vi "AlliGator Run XY Graph Python Function.vi"(6 "AlliGator Ctrl Refnums":T1, 8 "error in (no error)":errorcluster, 9 "Python Function Info":T9={"Script Path"=path "", "Function Name"="", "Function Parent Menu"="", "Function Input Parameters"=[], "Function Outputs"=[], "Function Doc String"="", "Function Display Name"="", "Function Target Type"=enum."Window Menu", "Function Target Window"="", "Parent Menu Location"="", "Item Menu Tag"="", "Is preceded by Separator"=FALSE}, 10 "Mouse Click Event Data":T13, 11 "data value reference in":refnum<data-value>) -> (0 "error out":errorcluster, 1 "Message":string, 3 "Data Value Reference out":refnum<data-value>)   [LabVIEW 2021, in "AlliGator Python Plugins.lvlib"]
doc: "Calls a XY Graph-associated python function."
uses:
  AlliGator Python Plugins.lvlib
  Graphs/XY Graph/XY Graph Mouse Click Event Data.ctl
  Graphs/XY Graph/XY Graph Refnum.ctl
  <vilib>/Utility/miscctls.llb/LVPoint32TypeDef.ctl
  AlliGator Python Function Information.ctl
  AlliGator Python Function Parameter Definition.ctl
  AlliGator Python Function Output Definition.ctl
  AlliGator Python Plugin Target Type.ctl
  AlliGator Internal Variables v2.ctl
  <vilib>/vision/Image Controls.llb/IMAQ Image.ctl
  AlliGator Gate Image Set.ctl
  AlliGator FLI Dataset Type.ctl
  AlliGator Data Series Type.ctl
  AlliGator Dataset Channel.ctl
  AlliGator Gate Arithmetic.ctl
  AlliGator Displayed Image.ctl
  Image/Named ROI Description.ctl
  AlliGator Decay Metadata v3.ctl
  AlliGator Decay Background Subtraction Info.ctl
  AlliGator Baseline Subtraction Method.ctl
  Graphs/XY Graph/XY Graph Plot Shift Parameters.ctl
  Graphs/XY Graph/XY Graph Plot Shift Method.ctl
  AlliGator Decay Extrapolation Parameters.ctl
  Phasor/Calibration Phasor (m, phi).ctl
  Phasor/Phasor Reference Series.ctl
  Phasor/Phasor Calibration Map v2.ctl
  Phasor/Phasor (g, s).ctl
  AlliGator Raw Phasor Plot Data v4.ctl
  Phasor/Phasor Standard Deviation Options.ctl
  AlliGator Phasor Multi-Harmonic Data.ctl
  Phasor/Phasor Harmonic Data.ctl
  AlliGator Decay Fit Options & Parameters v2.ctl
  Fits/IRF(X)PSED/Decay Fit Options v2.ctl
  Fits/Decay Convolution/Decay Model.ctl
  Fits/Residual Type.ctl
  Fits/IRF(X)PSED/Fit Weights Type.ctl
  Fits/Non-linear Fitting Method v2.ctl
  Fits/Fit Calculation Method.ctl
  Fits/Non-linear Fitting Algorithm.ctl
  AlliGator Decay Fit Parameter Constraints 2.ctl
  Fits/IRF(X)PSED/Decay Fit Parameters In List.ctl
  Fits/IRF(X)PSED/MLE Baseline Offset Type.ctl
  AlliGator Decay Preprocessing Parameters.ctl
  Fits/IRF(X)PSED/Decay Fit Parameters & Derived Quantities List.ctl
  AlliGator Ctrl Refnums.ctl
  AlliGator Other Ctrl Refnums.ctl
  AlliGator State Indicator.ctl
  AlliGator Phasor Plot Ctrl Refnums.ctl
  AlliGator Phasor Graph Ctrl Refnums.ctl
  Phasor/Phasor Calibration Type.ctl
  AlliGator Dataset Ctrl Refnums.ctl
  AlliGator Registered Events Ctrl Refnums.ctl
  AlliGator Image Histogram Control Refnums.ctl
  Histograms/Linear Histogram Options.ctl
  Histograms/Histogram Bin Option.ctl
  Histograms/Histogram Bin Position.ctl
  AlliGator Decay Fit Map Control Refnums.ctl
  AlliGator Variables List.ctl
  AlliGator Python Plugin Plot Data.ctl
  AlliGator Python Plugin Graph Data Input.ctl
  Graphs/Get Plot at Mouse Click (XY Graph)/Get Plot at Mouse Click [AAC].vi
  Graphs/XY Graph/XY Graph Add Multiplots with Names.vi
  Graphs/Graphs.lvlib
  Graphs/XY Graph/XY Graph Add-Ons.lvlib
  AlliGator Globals, Variables & Constants.lvlib
  Strings/Strings.lvlib
  Error/Error.lvlib
  AlliGator GUI.lvlib
  Phasor/Phasor.lvlib
  Image/Image.lvlib
  AlliGator Decay Preprocessing.lvlib
  AlliGator Phasor Graph.lvlib
  AlliGator Files.lvlib
  AlliGator Phasor Plot.lvlib
  AlliGator Source Image.lvlib
  Fits/Fits.lvlib
  AlliGator Decay Fit.lvlib
  AlliGator Decay Fit Parameter Map.lvlib
  AlliGator Settings.lvlib
  AlliGator Internal Variables.lvlib
  AlliGator Dual-Channel Datasets.lvlib
  Histograms/Histogram Window.lvlib
panel:
  out "Function Parameters String":string
  # "see the AlliGator License on the block diagram (Ctrl+E or Window:Show Block Diagram)"
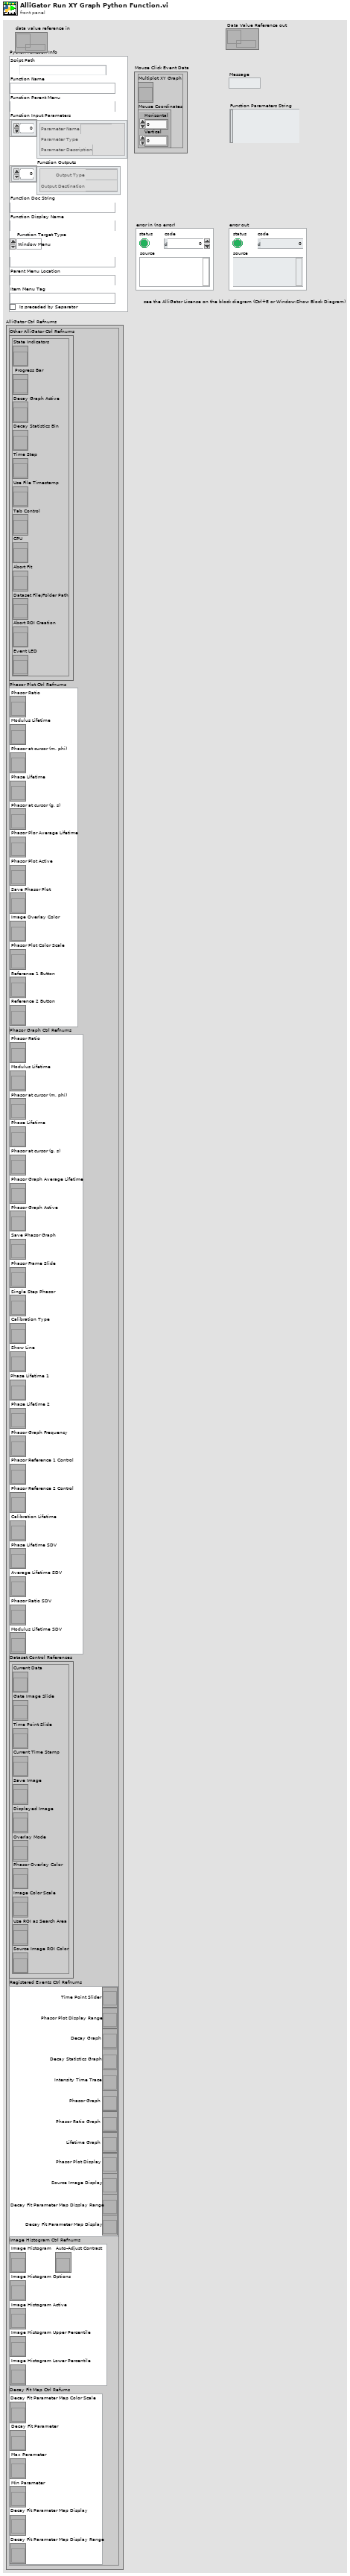
[diagram p1: front panel]
types:
  T1 = typedef "AlliGator GUI.lvlib/AlliGator Ctrl Refnums.ctl" = cluster{"Other AlliGator Ctrl Refnums":T2, "Phasor Plot Ctrl Refnums":T3, "Phasor Graph Ctrl Refnums":T4, "Dataset Control References":T5, "Registered Events Ctrl Refnums":T6, "Image Histogram Ctrl Refnums":T7, "Decay Fit Map Ctrl Refums":T8}
  T2 = typedef "AlliGator GUI.lvlib/AlliGator Other Ctrl Refnums.ctl" = cluster{"State Indicators":refnum<vi>, " Progress Bar":refnum<vi>, "Decay Graph Active":refnum<vi>, "Decay Statistics Bin":refnum<vi>, "Time Step":refnum<vi>, "Use File Timestamp":refnum<vi>, "Tab Control":refnum<vi>, "CPU":refnum<vi>, "Abort Fit":refnum<vi>, "Dataset File/Folder Path":refnum<vi>, "Abort ROI Creation":refnum<vi>, "Event LED":refnum<vi>}
  T3 = typedef "AlliGator GUI.lvlib/AlliGator Phasor Plot Ctrl Refnums.ctl" = cluster{"Phasor Ratio":refnum<vi>, "Modulus Lifetime":refnum<vi>, "Phasor at cursor (m, phi)":refnum<vi>, "Phase Lifetime":refnum<vi>, "Phasor at cursor (g, s)":refnum<vi>, "Phasor Plor Average Lifetime":refnum<vi>, "Phasor Plot Active":refnum<vi>, "Save Phasor Plot":refnum<vi>, "Image Overlay Color":refnum<vi>, "Phasor Plot Color Scale":refnum<vi>, "Reference 1 Button":refnum<vi>, "Reference 2 Button":refnum<vi>}
  T4 = typedef "AlliGator GUI.lvlib/AlliGator Phasor Graph Ctrl Refnums.ctl" = cluster{"Phasor Ratio":refnum<vi>, "Modulus Lifetime":refnum<vi>, "Phasor at cursor (m, phi)":refnum<vi>, "Phase Lifetime":refnum<vi>, "Phasor at cursor (g, s)":refnum<vi>, "Phasor Graph Average Lifetime":refnum<vi>, "Phasor Graph Active":refnum<vi>, "Save Phasor Graph":refnum<vi>, "Phasor Frame Slide":refnum<vi>, "Single Step Phasor":refnum<vi>, "Calibration Type":refnum<vi>, "Show Line":refnum<vi>, "Phase Lifetime 1":refnum<vi>, "Phase Lifetime 2":refnum<vi>, "Phasor Graph Frequency":refnum<vi>, "Phasor Reference 1 Control":refnum<vi>, "Phasor Reference 2 Control":refnum<vi>, "Calibration Lifetime":refnum<vi>, "Phase Lifetime SDV":refnum<vi>, "Average Lifetime SDV":refnum<vi>, "Phasor Ratio SDV":refnum<vi>, "Modulus Lifetime SDV":refnum<vi>}
  T5 = typedef "AlliGator GUI.lvlib/AlliGator Dataset Ctrl Refnums.ctl" = cluster{"Current Data":refnum<vi>, "Gate Image Slide":refnum<vi>, "Time Point Slide":refnum<vi>, "Current Time Stamp":refnum<vi>, "Save Image":refnum<vi>, "Displayed Image":refnum<vi>, "Overlay Mode":refnum<vi>, "Phasor Overlay Color":refnum<vi>, "Image Color Scale":refnum<vi>, "Use ROI as Search Area":refnum<vi>, "Source Image ROI Color":refnum<vi>}
  T6 = typedef "AlliGator GUI.lvlib/AlliGator Registered Events Ctrl Refnums.ctl" = cluster{"Time Point Slider":refnum<vi>, "Phasor Plot Display Range":refnum<vi>, "Decay Graph":refnum<vi>, "Decay Statistics Graph":refnum<vi>, "Intensity Time Trace":refnum<vi>, "Phasor Graph":refnum<vi>, "Phasor Ratio Graph":refnum<vi>, "Lifetime Graph":refnum<vi>, "Phasor Plot Display":refnum<vi>, "Source Image Display":refnum<vi>, "Decay Fit Parameter Map Display Range":refnum<vi>, "Decay Fit Parameter Map Display":refnum<vi>}
  T7 = typedef "AlliGator GUI.lvlib/AlliGator Image Histogram Control Refnums.ctl" = cluster{"Image Histogram":refnum<vi>, "Image Histogram Options":refnum<vi>, "Image Histogram Active":refnum<vi>, "Image Histogram Upper Percentile":refnum<vi>, "Image Histogram Lower Percentile":refnum<vi>, "Auto-Adjust Contrast":refnum<vi>}
  T8 = typedef "AlliGator Decay Fit Parameter Map.lvlib/AlliGator Decay Fit Map Control Refnums.ctl" = cluster{"Decay Fit Parameter Map Color Scale":refnum<vi>, "Decay Fit Parameter":refnum<vi>, "Max Parameter":refnum<vi>, "Min Parameter":refnum<vi>, "Decay Fit Parameter Map Display":refnum<vi>, "Decay Fit Parameter Map Display Range":refnum<vi>}
  T9 = typedef "AlliGator Python Plugins.lvlib/AlliGator Python Function Information.ctl" = cluster{"Script Path":path, "Function Name":string, "Function Parent Menu":string, "Function Input Parameters":T10[], "Function Outputs":T11[], "Function Doc String":string, "Function Display Name":string, "Function Target Type":T12, "Function Target Window":string, "Parent Menu Location":string, "Item Menu Tag":string, "Is preceded by Separator":bool}
  T10 = typedef "AlliGator Python Plugins.lvlib/AlliGator Python Function Parameter Definition.ctl" = cluster{"Parameter Name":string, "Parameter Type":string, "Parameter Description":string}
  T11 = typedef "AlliGator Python Plugins.lvlib/AlliGator Python Function Output Definition.ctl" = cluster{"Output Type":string, "Output Destination":string}
  T12 = typedef "AlliGator Python Plugins.lvlib/AlliGator Python Plugin Target Type.ctl" = enum16{"Undefined", "Window Menu", "Object Menu"}
  T13 = typedef "XY Graph Add-Ons.lvlib/XY Graph Mouse Click Event Data.ctl" = cluster{"Multiplot XY Graph":T14, "Mouse Coordinates":T15}
  T14 = typedef "XY Graph Add-Ons.lvlib/XY Graph Refnum.ctl" = refnum<vi>
  T15 = typedef "LVPoint32TypeDef.ctl" = cluster{"Horizontal":i32, "Vertical":i32}
  T16 = typedef "AlliGator Python Plugins.lvlib/AlliGator Python Plugin Graph Data Input.ctl" = cluster{"Graph_Name":string, "Plots":T17[], "Reference_Decay":T17}
  T17 = typedef "AlliGator Python Plugins.lvlib/AlliGator Python Plugin Plot Data.ctl" = cluster{"Plot_Name":string, "X_Array":dbl[], "Y_Array":dbl[]}
  T18 = typedef "AlliGator Globals, Variables & Constants.lvlib/AlliGator Variables List.ctl" = enum16{"---- GUI ----", "Initialization Status", "State Indicators Refnum", "Original AlliGator Menu Items", "Current Action Loop State", "Script in progress", "Playback", "Loop Playback", "Search ROI Used", "Search ROI", "Decay Graph Max Legend Size", "Intensity Graph Max Legend Size", "Decay Statistics Graph Max Legend Size", "Phasor Graph Max Legend Size", "Phasor Ratio Graph Max Legend Size", "Lifetime Graph Max Legend Size", "---- Files ----", "Export Dataset Frames as Individual Files", "Show Batch Export Help Balloons", "Frames in Dataset", "ptu File Frame Start Indices", "Current Frame in Dataset", "Current Frame Timestamp", "------ Python Plugins ------", "Python Plugins Information", "Python Session", "Valid Python Session?", "---- Source Image ----", "Dataset Loaded", "Dataset Metadata", "Dataset Channel", "Dataset Data Description", "Background Dataset Metadata", "Background Dataset Channel", "Background Dataset Data Description", "Background File Subtraction", "Background File Path", "Background File Pile-up Correction", "Background File Pixel Well Capacity", "Background File Scaling Factor", "Source Image ROIs", "Current Source Image ROI", "Source Image ROI Event Refnum", "X_Source Image Display Range", "X_Source Image Palette Information", "Source Image Palette List", "Source Image Scale", "Current Dataset Load Settings", "Source Image:ROI Overlay Color", "---- Image Profile Window ----", "Image Profile:Overlay ROI in Source Image", "Image Profile Window Event Refnum", "Image Profile:IntensityType", "Image Profile:Intensity Average Type", "Image Profile:Intensity-weighted SDV", "Image Profile:Box Profile Type", "Image Profile Window Open", "Image Profile:Plotted Fit Parameter", "X_Type of Displayed Image", "X_Time Gate Slider", "Dataset Path", "Source Image Overlay to Erase", "Is Displayed Image Accumulated", "White Light Image Modified", "Mask Image Modified", "Macrotime Gate Separation", "------ Phasor Graph -------", "Phasor Graph:Show Line", "---- Phasor Plot ---", "Phasor Plot Parameters Changed", "FLI Dataset Modified since last Phasor Plot Calculation", "Phasor Harmonics Data", "Selected Phasor Harmonics", "Phasor Harmonic Manager Event Refnum", "Phasor Plot ROIs", "Current Phasor Plot ROI", "Phasor Plot ROI Event Refnum", "Phasor Plot Image Reference Points", "Phasor Plot Computed", "Phasor Plot Palette Information", "Phasor Plot Palette List", "Phasor Ratio Palette Information", "Phasor Ratio Palette List", "Phasor Image Scale", "Phasor Plot Image Overlay to Erase", "Phasor Plot Image Elements to Update", "Current Phasor Plot Calculation Parameters", "Current Phasor Calibration Options", "Reset Cumulated Phasor Plot", "Phasor Ratio Reference 1", "Phasor Ratio Lifetime Reference 1", "Phasor Ratio Reference 1 Frequency", "Phasor Ratio Reference 2", "Phasor Ratio Lifetime Reference 2", "Phasor Ratio Reference 2 Frequency", "---- Decay Analysis ----", "Number of Selected Decays to Fit", "LS Fit Results", "LAR Fit Results", "BS Fit Results", "Last Decay Max - Min", "Best Fit Parameters", "Best Fit Parameter Names", "Actual Size X", "Actual Size Y", "Binning X", "Binning Y", "Actual # Gates", "Dataset Number", "Gates to...", "Gates Skipped", "Gates to keep", "Gate Step", "Gate Separation", "Reversed Gates", "Pile-up Correction", "Pixel Well Capacity", "Background Subtracted", "Background Subtraction Method", "Background Definition Range", "Background File (deprecated)", "Number of Dataset Accumulated", "Array of Accumulated Dataset Paths", "Do Averaged Datasets", "Destination File Path", "Process Plot Target", "Use 1/D as Phasor Frequency", "---- Decay Fit Parameter Map -----", "Decay Fit Parameter Map Palette Information", "Decay Fit Parameter Map Palette List", "Local Decay Graph Window Event Refnum", "------- Local Decay Window ---------", "Use normalized IRF for convolution", "----- Miscellaneous ----", "Skippable Dialog Windows Status"}
  T19 = typedef "AlliGator Python Plugins.lvlib/AlliGator Type of Plot Data.ctl" = enum16{"Single Plot", "Selected Plots", "All Plots"}
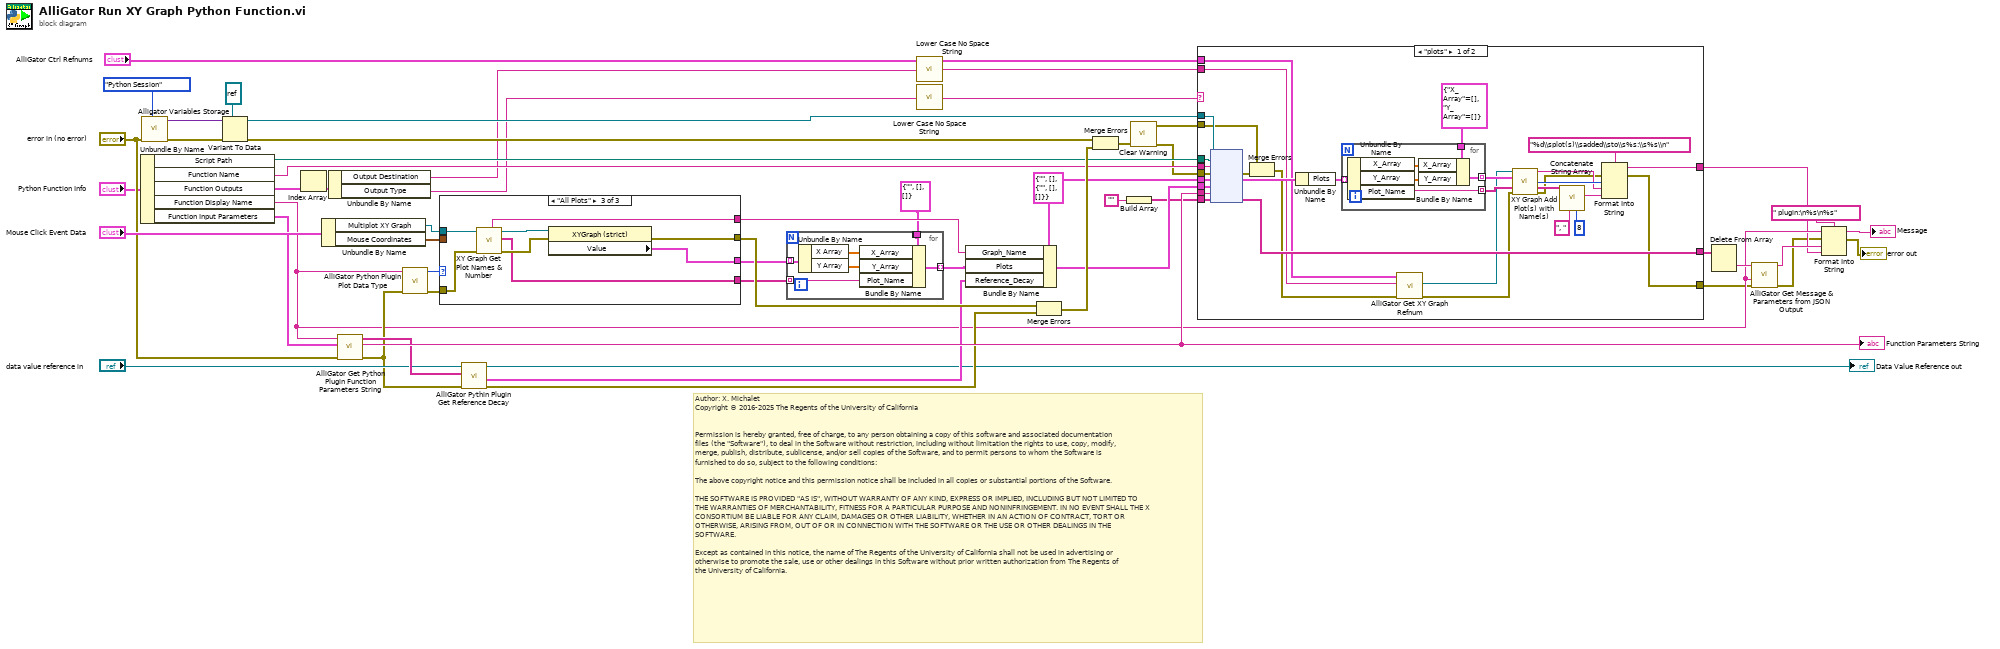
[diagram p0: block diagram]
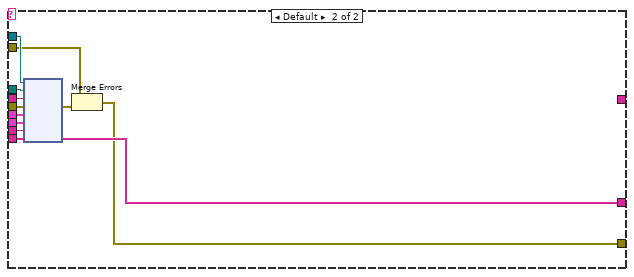
[diagram p2: hidden frame]
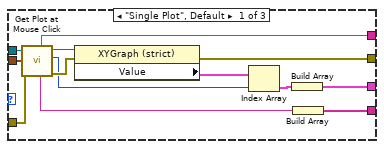
[diagram p3: hidden frame]
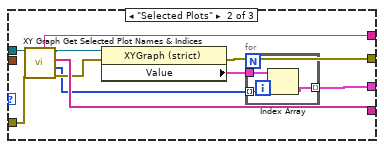
[diagram p4: hidden frame]
diagram:
  w21 = T16 {"Graph_Name"="", "Plots"=[], "Reference_Decay"={"Plot_Name"="", "X_Array"=[], "Y_Array"=[]}} ("Graph Plugin Data")
  # "Author: X. Michalet\nCopyright © 2016-2025 The Regents of the University of California\n \n\nPermission is hereby granted, free of charge, to any person obtaining a copy of this software and associated documentation files (the \"Software\"), to deal in the Software without restriction, including without limitation the rights to use, copy, modify, merge, publish, distribute, sublicense, and/or sell copies of the Software, and to permit persons to whom the Software is furnished to do so, subject to the following conditions:\n\nThe above copyright notice and this permission notice shall be included in all copies or substantial portions of the Software.\n\nTHE SOFTWARE IS PROVIDED \"AS IS\", WITHOUT WARRANTY OF ANY KIND, EXPRESS OR IMPLIED, INCLUDING BUT NOT LIMITED TO THE WARRANTIES OF MERCHANTABILITY, FITNESS FOR A PARTICULAR PURPOSE AND NONINFRINGEMENT. IN NO EVENT SHALL THE X CONSORTIUM BE LIABLE FOR ANY CLAIM, DAMAGES OR OTHER LIABILITY, WHETHER IN AN ACTION OF CONTRACT, TORT OR OTHERWISE, ARISING FROM, OUT OF OR IN CONNECTION WITH THE SOFTWARE OR THE USE OR OTHER DEALINGS IN THE SOFTWARE.\n\nExcept as contained in this notice, the name of The Regents of the University of California shall not be used in advertising or otherwise to promote the sale, use or other dealings in this Software without prior written authorization from The Regents of the University of California."
  n1 = Unbundle By Name("Python Function Info") -> ("Script Path"=w32:path, "Function Name"=w28:string, "Function Outputs"=w11:T11[], "Function Display Name"=w16:string, "Function Input Parameters"=w31:T10[])
  n2 = call "Alligator Variables Storage.vi"("AlliGator Variable"=AlliGator_Variables_List."Python Session" ("Alligator Variable"), "Error In"="error in (no error)") -> ("Error Out"=w47:errorcluster, "Data out"=w45:variant)  [unwired: 7 in, 1 out]
  n3 = Variant To Data(error in=w47, type=refnum<k35> refnum ("session in"), Variant=w45) -> (data=w43:refnum<k35>, error out=w46:errorcluster)
  n4 = Index Array(array=w11) -> (element=w10:T11)  [unwired: 1 in]
  n5 = Unbundle By Name("Mouse Click Event Data") -> ("Multiplot XY Graph"=w53:T14, "Mouse Coordinates"=w52:T15)
  n6 = Unbundle By Name(w10) -> ("Output Destination"=w5:string, "Output Type"=w8:string)
  n7 = call "AlliGator Get Python Plugin Function Parameters String.vi"("error in (no error)"="error in (no error)", "Function Parameters"=w31, "Function Display Name"=w16) -> ("error out"=w25:errorcluster, "Function Parameters JSON String"=w42:string, "Parameter Names Not Found"=w27:string[])  [unwired: 6 in]
  "Function Parameters String" <- w42
  n8 = call "AlliGator Python Plugin Plot Data Type.vi"("error in (no error)"=w25, "Function Name"=w16) -> ("error out"=w40:errorcluster, "Type of Plot Data"=w41:T19)  [unwired: 8 in]
  n9 = case shown="\"All Plots\"" w41 {
    tunnel: w53 -> [w63 w77 w86]
    tunnel: w52 -> [w62 _ _]
    tunnel: [w61 w68 w87] -> w39
    tunnel: [w58 w74 w81] -> w35
    tunnel: w40 -> [w59 w76 w85]
    tunnel: [w57 w69 w88] -> w36
    tunnel: [w56 w75 w82] -> w37
    frame "Single Plot", Default {
      n10 = call-poly "Get Plot at Mouse Click.vi"("error in (no error)"=w59, "Mouse Click Coordinates"=w62, "XYGraph Ref"=w63) -> ("error out"=w66:errorcluster, "Plot at Coordinates"=w64:i32, "XYGraph Ref"=w67:T14, "Plot Name"=w60:string, "Graph Name"=w56:string)  [unwired: 2 in, 2 out]
      n11 = property class="XYGraph (strict)"(reference=w67, error in=w66) -> (error out=w61:errorcluster, "Value"=w65:cluster{"X Array":dbl[], "Y Array":dbl[]}[])  [unwired: 1 out]
      n12 = Index Array(array=w65, index=w64) -> (element=w55:cluster{"X Array":dbl[], "Y Array":dbl[]})
      n13 = Build Array(w55) -> (w57:cluster{"X Array":dbl[], "Y Array":dbl[]}[])
      n14 = Build Array(w60) -> (w58:string[])
    }
    frame "Selected Plots" {
      n15 = call "XY Graph Get Selected Plot Names & Indices.vi"("error in (no error)"=w76, "XYGraph in"=w77) -> ("error out"=w73:errorcluster, "Selected Plots"=w71:i32[], "Selected Plot Names"=w74:string[], "XYGraph out"=w72:T14, "Graph Name"=w75:string)  [unwired: 5 in]
      n16 = property class="XYGraph (strict)"(reference=w72, error in=w73) -> (error out=w68:errorcluster, "Value"=w70:cluster{"X Array":dbl[], "Y Array":dbl[]}[])  [unwired: 1 out]
      n17 = for {
        tunnel: w71 -> [w80] mode=indexing
        tunnel: w70 -> [w79]
        tunnel: [w78] -> w69 mode=indexing
        n18 = Index Array(array=w79, index=w80) -> (element=w78:cluster{"X Array":dbl[], "Y Array":dbl[]})
      }
    }
    frame "All Plots" {
      n19 = call "XY Graph Get Plot Names & Number.vi"("error in (no error)"=w85, "XYGraph in"=w86) -> ("error out"=w84:errorcluster, "Plot Names"=w81:string[], "XYGraph out"=w83:T14, "Graph Name"=w82:string)  [unwired: 4 in, 2 out]
      n20 = property class="XYGraph (strict)"(reference=w83, error in=w84) -> (error out=w87:errorcluster, "Value"=w88:cluster{"X Array":dbl[], "Y Array":dbl[]}[])  [unwired: 1 out]
    }
  }
  n21 = call "AlliGator Pythin Plugin Get Reference Decay.vi"("error in (no error)"=w25, "AlliGator Parameter Names in"=w27, "Data Value Reference in"="data value reference in") -> ("error out"=w24:errorcluster, "Reference Decay"=w23:T17, "Data Value Reference out"=→"Data Value Reference out":refnum<data-value>)  [unwired: 4 in, 2 out]
  n22 = for {
    tunnel: w35 -> [w94] mode=indexing
    tunnel: [w93] -> w20 mode=indexing
    tunnel: [w89] -> _
    tunnel: w36 -> [w92] mode=indexing
    tunnel: T17 {"Plot_Name"="", "X_Array"=[], "Y_Array"=[]} ("Plugin Plot Data") -> [w89]
    n23 = Unbundle By Name(w92) -> ("X Array"=w91:dbl[], "Y Array"=w90:dbl[])
    n24 = Bundle By Name(cluster=w89, "X_Array"=w91, "Y_Array"=w90, "Plot_Name"=w94) -> (w93:T17)
  }
  n25 = call "Lower Case No Space String.vi"("String"=w5) -> ("Lower Case No Space String"=w4:string)
  n26 = call "Lower Case No Space String.vi"("String"=w8) -> ("Lower Case No Space String"=w7:string)
  n27 = Bundle By Name(cluster=w21, "Graph_Name"=w37, "Plots"=w20, "Reference_Decay"=w23) -> (w22:T16)
  n28 = Merge Errors(w39, w24) -> (w38:errorcluster)
  n29 = Merge Errors(w46, w38) -> (w14:errorcluster)
  n30 = Build Array("") -> (w17:string[])
  n31 = call "Clear Warning.vi"("error in (no error)"=w14) -> ("cleared warning or error dup"=w13:errorcluster, "error in (dup)"=w12:errorcluster)  [unwired: 9 in]
  n32 = case shown="\"plots\"" w7 {
    tunnel: w43 -> [w125 w143]
    tunnel: w42 -> [w124 w142]
    tunnel: w32 -> [w120 w141]
    tunnel: [w119 w140] -> w30
    tunnel: w28 -> [w117 w138]
    tunnel: w22 -> [w113 w137]
    tunnel: w21 -> [w112 w136]
    tunnel: w17 -> [w109 w135]
    tunnel: w13 -> [w108 w134]
    tunnel: w12 -> [w107 w133]
    tunnel: [w101 _] -> w9
    tunnel: [w100 w132] -> w6
    tunnel: w4 -> [w97 _]
    tunnel: "AlliGator Ctrl Refnums" -> [w95 _]
    frame "plots" {
      n33 = node(w125, w120, w117, w108, w112, w113, w124, w109) -> (w118:errorcluster, w123:T16, w119:string[])  [unwired: 2 in, 3 out]
      n34 = Merge Errors(w107, w118) -> (w99:errorcluster)
      n35 = Unbundle By Name(w123) -> ("Plots"=w110:T17[])
      n36 = for {
        tunnel: w110 -> [w131] mode=indexing
        tunnel: [w130] -> w121 mode=indexing
        tunnel: cluster{"X_Array":dbl[], "Y_Array":dbl[]} {"X_Array"=[], "Y_Array"=[]} -> [w128]
        tunnel: [w126] -> w122 mode=indexing
        n37 = Unbundle By Name(w131) -> ("X_Array"=w129:dbl[], "Y_Array"=w127:dbl[], "Plot_Name"=w130:string)
        n38 = Bundle By Name(cluster=w128, "X_Array"=w129, "Y_Array"=w127) -> (w126:cluster{"X_Array":dbl[], "Y_Array":dbl[]})
      }
      n39 = call "AlliGator Get XY Graph Refnum.vi"("error in (no error)"=w99, "XY Graph Name"=w97, "AlliGator Ctrl Refnums"=w95) -> ("error out"=w98:errorcluster, "XY Graph reference"=w96:T14)  [unwired: 7 in]
      n40 = call-poly "XY Graph Add Plot(s) with Name(s).vi"("XYGraph in"=w96, "Array of Plots"=w122, "Array of Plot Names (\"Plot\")"=w121, "error in (no error)"=w98) -> ("XY Graph Caption"=w104:string, "Number of Plots Added"=w105:i32, "Added Plot Names"=w116:string[], "error out"=w102:errorcluster)  [unwired: 7 in, 1 out]
      n41 = call "Concatenate String Array.vi"("Max Number of Elements (None: -1)"=8, "Separator (TAB)"=", ", "String Array"=w116) -> ("Formatted String"=w103:string)  [unwired: 8 in]
      n42 = Format Into String(format string="%d\\splot(s)\\sadded\\sto\\s%s:\\s%s\\n", error in=w102, w105, w104, w103) -> (resulting string=w101:string, error out=w100:errorcluster)  [unwired: 1 in]
    }
    frame Default {
      n43 = node(w143, w141, w138, w134, w136, w137, w142, w135) -> (w139:errorcluster, w140:string[])  [unwired: 3 in, 3 out]
      n44 = Merge Errors(w133, w139) -> (w132:errorcluster)
    }
  }
  n45 = Delete From Array(array=w30) -> (deleted portion=w29:string)  [unwired: 2 in, 1 out]
  n46 = call "AlliGator Get Message & Parameters from JSON Output.vi"("error in (no error)"=w6, "Function Display Name"=w16, "<JSON>"=w29) -> ("error out"=w1:errorcluster, "Notebook Message"=w15:string)  [unwired: 7 in]
  n47 = Format Into String(format string=" plugin:\n%s\n%s", initial string=w16, error in=w1, w15, w9) -> (resulting string=→"Message":string, error out=→"error out":errorcluster)
